vi "ClosePowerSupply.vi"(1 "IVI Logical Name":refnum<k15>) -> (0 "error out":errorcluster {"code" format="%.0x"})   [LabVIEW 2013]
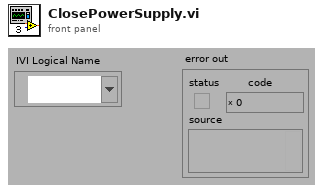
[diagram p1: front panel]
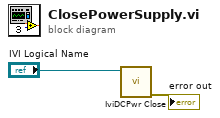
[diagram p0: block diagram]
diagram:
  n1 = call <vilib>:"IviDCPwr Close.vi"("instrument handle"="IVI Logical Name") -> ("error out"=→"error out":errorcluster)  [unwired: 1 in, 9 out]
